vi "sinusiodal waveform generation.vi"() -> ()   [LabVIEW 2025]
panel:
  out "sinusodial output":dynamicdata(graph)
  in  "phase":dbl
  in  "offset":dbl
  in  "frequency":dbl
  in  "amplitude":dbl
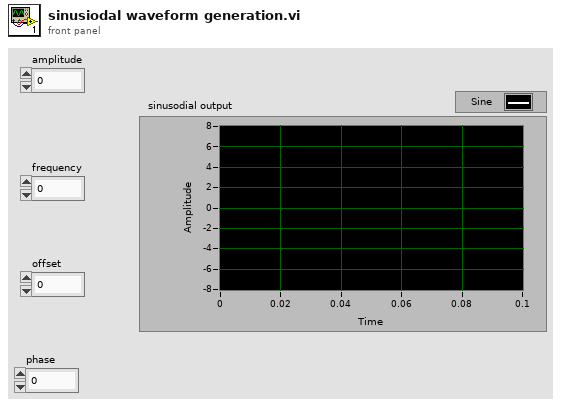
[diagram p1: front panel]
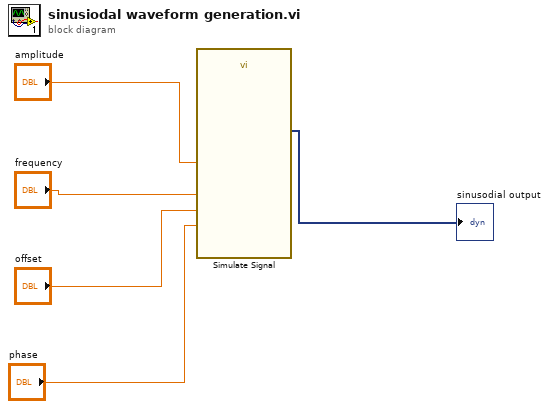
[diagram p0: block diagram]
diagram:
  n1 = call "Simulate Signal"("Offset"="offset", "Frequency"="frequency", "Amplitude"="amplitude", "Phase"="phase") -> ("Sine"=→"sinusodial output":dynamicdata)  [unwired: 10 in, 1 out]
